vi "CSVReadMap.vi"(11 "file path (dialog if empty)":path=path "C:/Projects/DTC/TestStand/v5 input registers/sequences/MLX90327.csv") -> (1 "Address Status":i32[](array[numeric]) format="%04x", 2 "Final Val":i32[](array[numeric]) format="%04x", 3 "Initial_Val":u32[](array[numeric]) format="%04x")   [LabVIEW 2020]
uses:
  <vilib>/Utility/file.llb/Read Delimited Spreadsheet (string).vi
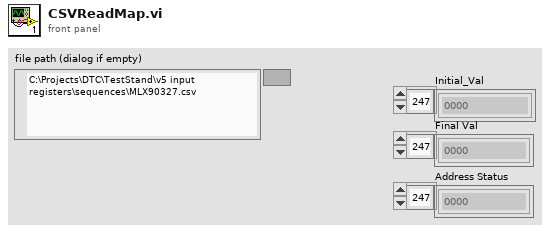
[diagram p1: front panel]
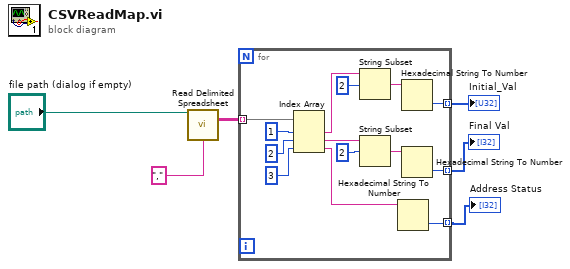
[diagram p0: block diagram]
diagram:
  n1 = call-poly <vilib>:"Read Delimited Spreadsheet.vi"("file path (dialog if empty)"="file path (dialog if empty)", "delimiter (\\t)"="," ("delimiter (\\t)")) -> ("all rows"=w4:string[][])  [unwired: 8 in, 5 out]
  n2 = for {
    tunnel: w4 -> [w20] mode=indexing
    tunnel: [w16] -> w3 mode=indexing
    tunnel: [w10] -> w2 mode=indexing
    tunnel: [w8] -> w1 mode=indexing
    n3 = Index Array(array=w20, index #1=1 ("index"), index #2=2 ("index"), index #3=3 ("index")) -> (element #1=w15:string, element #2=w13:string, element #3=w7:string)
    n4 = String Subset(string=w15, offset (0)=2) -> (substring=w14:string)  [unwired: 1 in]
    n5 = String Subset(string=w13, offset (0)=2) -> (substring=w11:string)  [unwired: 1 in]
    n6 = Hexadecimal String To Number(string=w7) -> (number=w8:u32)  [unwired: 2 in, 1 out]
    n7 = Hexadecimal String To Number(string=w14) -> (number=w16:u32)  [unwired: 2 in, 1 out]
    n8 = Hexadecimal String To Number(string=w11) -> (number=w10:u32)  [unwired: 2 in, 1 out]
  }
  "Initial_Val" <- w3
  "Final Val" <- w2
  "Address Status" <- w1
